vi "SET_TAPE_MEASURE_SPEED.vi"(10 "argv":string[](array[string]), 11 "args":u8) -> ()   [LabVIEW 2014]
uses:
  Robot Global Data.vi
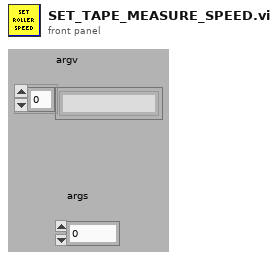
[diagram p1: front panel]
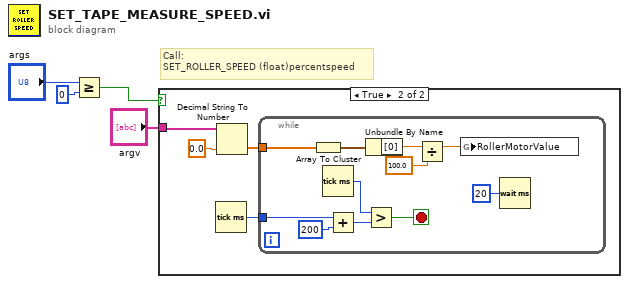
[diagram p0: block diagram]
diagram:
  # "Call:\nSET_ROLLER_SPEED (float)percentspeed"
  n1 = Greater Or Equal?(x="args", y=u8 0) -> (x >= y?=w4:bool)
  n2 = case shown="True" w4 {
    tunnel: "argv" -> [_ w5]
    frame False {
    }
    frame True {
      n3 = Tick Count (ms)() -> (millisecond timer value=w6:u32)
      n4 = Decimal String To Number(string=w5, default (0L)=0.0 ("default (0 I32)")) -> (number=w7:dbl[])  [unwired: 2 out]
      n5 = while {
        tunnel: w7 -> [w19]
        tunnel: w6 -> [w17]
        stop <- w13 stop-if-true
        n6 = Array To Cluster(array=w19) -> (cluster=w18:cluster{"[0]":dbl, "[1]":dbl})
        n7 = Tick Count (ms)() -> (millisecond timer value=w15:u32)
        n8 = Add(x=w17, y=u32 200) -> (x+y=w14:u32)
        n9 = Unbundle By Name(w18) -> ("[0]"=w11:dbl)
        n10 = Greater?(x=w15, y=w14) -> (0:w13:bool)
        n11 = Divide(x=w11, y=100.0) -> (x/y=w10:dbl)
        n12 = global write "Robot Global Data.vi" "RollerMotorValue"(w10) -> ()
        n13 = Wait (ms)(milliseconds to wait=u32 20) -> ()  [unwired: 1 out]
      }
    }
  }
